vi "Handle Error.vi"(8 "error in (no error)":errorcluster, 11 "Simulated User Console Actor in":refnum<class "Simulated User Console Actor.lvclass">) -> (0 "error out":errorcluster, 2 "stop actor?":bool=TRUE, 3 "Simulated User Console Actor out":refnum<class "Simulated User Console Actor.lvclass">)   [LabVIEW 2019, in "Simulated User Console Actor.lvlib" / "Simulated User Console Actor.lvclass"]
doc: "(<B>Filename</B>: Actor Framework.lvlib:Actor.lvclass:Handle Error.vi)\n\nDefines how the actor handles an error that occurred while processing a message. By default, this method does nothing except stop the actor."
uses:
  Simulated User Console Actor.lvclass
  C:/Program Files (x86)/National Instruments/LabVIEW 2019/vi.lib/ActorFramework/Actor/Actor.lvclass
  ATM Controller/ATM Controller/Error Level.ctl
  <vilib>/ActorFramework/Actor/Actor.lvclass/Actor.ctl
  ATM Controller/ATM Controller Messages/Centrialize Error Handler Msg/Centrialize Error Handler Msg.lvclass/Centrialize Error Handler Msg.ctl
  <vilib>/ActorFramework/Message Enqueuer/Message Enqueuer.lvclass/Message Enqueuer.ctl
  <vilib>/ActorFramework/Message Enqueuer/Enqueue.vi
  ATM Controller/ATM Controller Messages/Centrialize Error Handler Msg/Centrialize Error Handler Msg.lvclass
  C:/Program Files (x86)/National Instruments/LabVIEW 2019/vi.lib/ActorFramework/Message/Message.lvclass
  <vilib>/ActorFramework/Message Priority Queue/Priority Enqueue.vi
  User Console Actor/User Console Actor/User Console Actor.lvclass
  <vilib>/ActorFramework/Actor/Actor.lvclass
  ATM Controller/ATM Controller/ATM Controller.lvclass
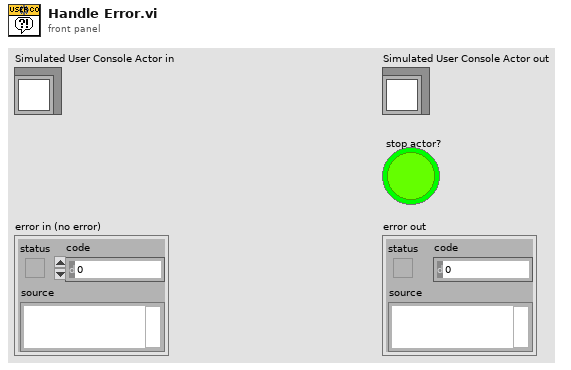
[diagram p1: front panel]
types:
  T1 = typedef "ATM Controller.lvlib/ATM Controller.lvclass/Error Level.ctl" = enum16{"Console Error", "Sensor Interface Error", "Process Step Error"}
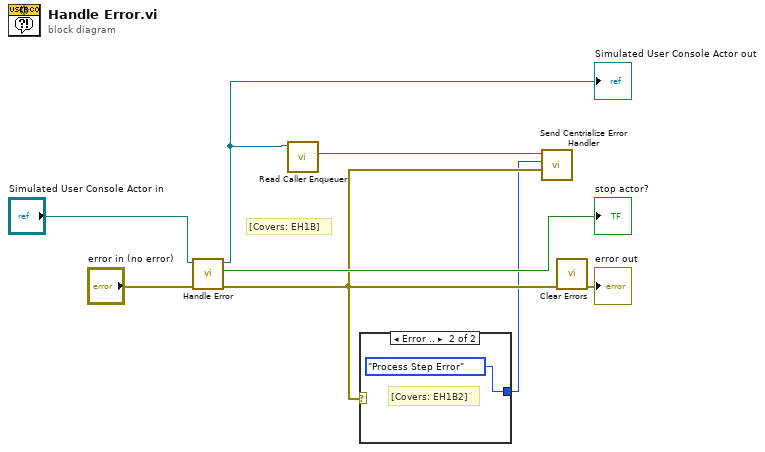
[diagram p0: block diagram]
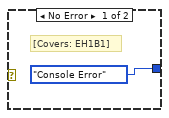
[diagram p2: hidden frame]
diagram:
  # "[Covers: EH1B]"
  n1 = call-parent "Handle Error.vi"("error in (no error)"="error in (no error)", "Actor in"="Simulated User Console Actor in") -> ("error out"=w2:errorcluster, "stop actor?"=→"stop actor?":bool, "Actor out"=w4:refnum<class "Simulated User Console Actor.lvclass">)  [unwired: 7 in]
  "Simulated User Console Actor out" <- w4
  n2 = call <vilib>:"Read Caller Enqueuer.vi"("Actor"=w4) -> ("Caller Enqueuer"=w5:refnum<class "Message Enqueuer.lvclass">)  [unwired: 10 in]
  n3 = case shown="Error .." w2 {
    tunnel: [Error_Level."Console Error" ("Error Level") Error_Level."Process Step Error" ("Error Level")] -> w1
    frame No Error {
      # "[Covers: EH1B1]"
    }
    frame Error {
      # "[Covers: EH1B2]"
    }
  }
  n4 = call "Send Centrialize Error Handler.vi"("Error"=w2, "Error Level"=w1, "Message Enqueuer"=w5) -> ()  [unwired: 7 in, 2 out]
  n5 = call <vilib>:"Clear Errors.vi"("error in (no error)"=w2) -> ("error out"=→"error out":errorcluster)  [unwired: 5 in, 1 out]
